vi "BoldFirstRow.vi"(8 "error in (no error)":errorcluster, 10 "Bold first row?":bool=TRUE, 11 "Playlist Ref":refnum<vi>) -> (0 "error out":errorcluster)   [LabVIEW 2015]
uses:
  <vilib>/Utility/miscctls.llb/LVRowAndColumnTypeDef.ctl
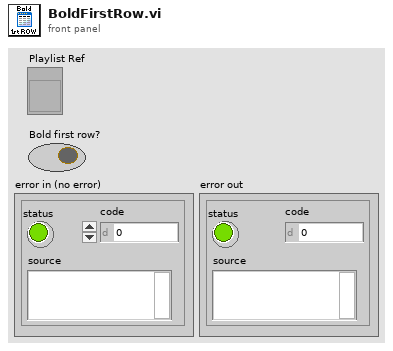
[diagram p1: front panel]
types:
  T1 = typedef "LVRowAndColumnTypeDef.ctl" = cluster{"Row":i32, "Column":i32}
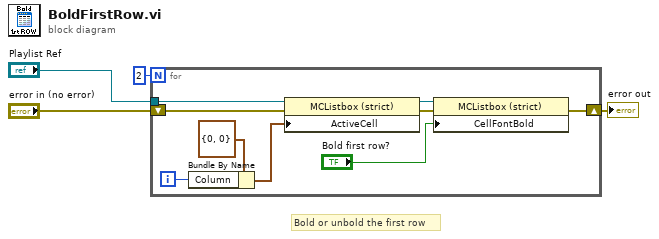
[diagram p0: block diagram]
diagram:
  # "Bold or unbold the first row"
  n1 = for {
    N: 2 -> [_]
    tunnel: "Playlist Ref" -> [w9]
    shift-right: [w12] -> w4
    shift-left: "error in (no error)" -> [w8]
    i -> [w6]
    n2 = Bundle By Name(cluster=T1 {"Row"=0, "Column"=0} ("Active Cell:Active Cell"), "Column"=w6) -> (w5:T1)
    n3 = property class="MCListbox (strict)"(reference=w9, error in=w8, "ActiveCell"=w5) -> (reference out=w10:refnum<vi>, error out=w11:errorcluster)
    n4 = property class="MCListbox (strict)"(reference=w10, error in=w11, "CellFontBold"="Bold first row?") -> (error out=w12:errorcluster)  [unwired: 1 out]
  }
  "error out" <- w4
